vi "Get Param (Map).vi"(8 "error in (no error)":errorcluster, 9 "Default":variant, 10 "Name":string, 11 "Request in":refnum<class "Request.lvclass">) -> (0 "error out":errorcluster, 1 "Value":variant, 2 "Found?":bool, 3 "Request out":refnum<class "Request.lvclass">)   [LabVIEW 2023, in "Request.lvclass"]
uses:
  Request.lvclass
  Request.lvclass/Request.ctl
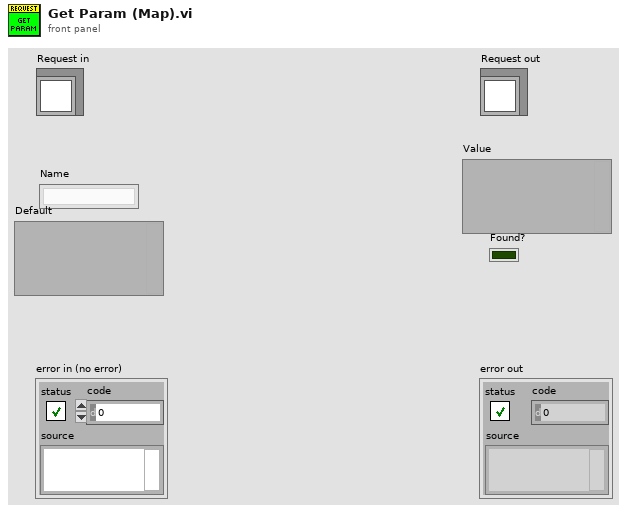
[diagram p1: front panel]
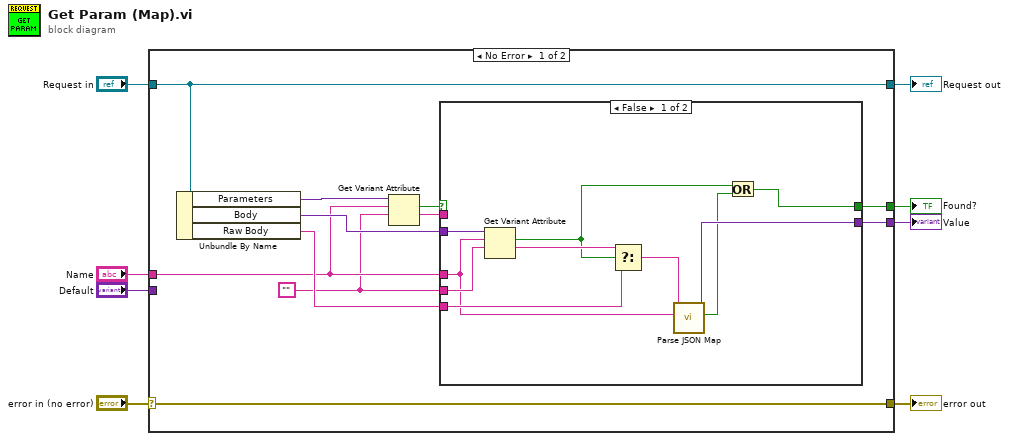
[diagram p0: block diagram]
diagram:
  n1 = case shown="No Error" "error in (no error)" {
    selector: "error in (no error)" -> [w19 w32]
    tunnel: [w19 w32] -> w7
    tunnel: [w18 w33] -> w5
    tunnel: "Request in" -> [w18 w33]
    tunnel: [w13 _] -> w4
    tunnel: "Name" -> [w10 _]
    tunnel: [w12 _] -> w2
    tunnel: "Default" -> [_ _]
    frame No Error {
      w9 = ""
      n2 = Unbundle By Name(w18) -> ("Parameters"=w17:variant, "Body"=w15:variant, "Raw Body"=w11:string)
      n3 = Get Variant Attribute(Variant=w17, name=w10, default value (empty Variant)=w9) -> (found=w16:bool, value=w14:string)  [unwired: 1 in, 2 out]
      n4 = case shown="False" w16 {
        selector: w16 -> [_ w30]
        tunnel: w15 -> [w29 _]
        tunnel: w14 -> [_ w31]
        tunnel: [w24 w31] -> w13
        tunnel: [w21 w30] -> w12
        tunnel: w11 -> [w26 _]
        tunnel: w9 -> [w28 _]
        tunnel: w10 -> [w20 _]
        frame False {
          n5 = Get Variant Attribute(Variant=w29, name=w20, default value (empty Variant)=w28) -> (found=w23:bool, value=w27:string)  [unwired: 1 in, 2 out]
          n6 = Select(t=w27, s=w23, f=w26) -> (s? t:f=w25:string)
          n7 = call "Parse JSON Map.vi"("Name"=w20, "JSON"=w25) -> ("Found?"=w22:bool, "Map"=w24:variant)  [unwired: 8 in]
          n8 = Or(x=w23, y=w22) -> (x .or. y?=w21:bool)
        }
        frame True {
        }
      }
    }
    frame Error {
    }
  }
  "error out" <- w7
  "Request out" <- w5
  "Value" <- w4
  "Found?" <- w2
